vi "Initialize Tx Transfers.vi"(8 "error in (no error)":errorcluster, 10 "Tx Transfer configurations":T2[](array[typedef]) {"channels"."string offset" format="%d bytes"}, 11 "UDP Transceiver in":refnum<class "UDP Transceiver.lvclass">) -> (0 "error out":errorcluster, 1 "max buffer size":u64, 2 "Tx Transfer parameters":T1[](array[typedef]), 3 "UDP Transceiver out":refnum<class "UDP Transceiver.lvclass">)   [LabVIEW 2017, in "UDP.lvlib" / "UDP Transceiver.lvclass"]
uses:
  UDP Transceiver.lvclass
  Builds/Data Sharing Framework/Current/Core/DSF Core.lvlibp/Typedefs/DSF Engine Transfer Configuration.ctl
  Builds/Data Sharing Framework/Current/Core/DSF Core.lvlibp/Typedefs/DSF Byte Order.ctl
  Builds/Data Sharing Framework/Current/Core/DSF Core.lvlibp/Typedefs/DSF Settings Info.ctl
  Builds/Data Sharing Framework/Current/Core/DSF Core.lvlibp/Typedefs/DSF Engine Channel Configuration.ctl
  Builds/Data Sharing Framework/Current/Core/DSF Core.lvlibp/Typedefs/DSF Data Type.ctl
  Transfer Tx Parameters.ctl
  Builds/Data Sharing Framework/Current/Core/DSF Core.lvlibp/Typedefs/DSF Buffer Type.ctl
  UDP Transceiver.lvclass/UDP Transceiver.ctl
  Builds/Data Sharing Framework/Current/Core/DSF Core.lvlibp/Classes/Configuration/Required Buffer Size (Transfer).vi
  UDP Invalid Setting.vi
  Builds/Data Sharing Framework/Current/Core/DSF Core.lvlibp/Classes/Configuration/Configuration Session.lvclass
  Builds/Data Sharing Framework/Current/Core/DSF Core.lvlibp
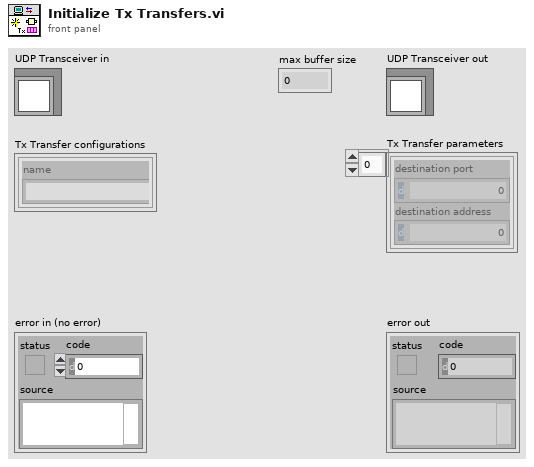
[diagram p1: front panel]
types:
  T1 = typedef "UDP.lvlib/UDP Transceiver.lvclass/Transfer Tx Parameters.ctl" = cluster{"destination port":u16, "destination address":u32}
  T2 = typedef "DSF Core.lvlibp/DSF Engine Transfer Configuration.ctl" = cluster{"name":string, "byte order":T3, "settings":T4, "channels":T5[]}
  T3 = typedef "DSF Core.lvlibp/DSF Byte Order.ctl" = enum8{"big-endian", "little-endian"}
  T4 = typedef "DSF Core.lvlibp/DSF Settings Info.ctl" = cluster{"component":string, "name":string, "values":cluster{"key":string, "value":string}[]}[]
  T5 = typedef "DSF Core.lvlibp/DSF Engine Channel Configuration.ctl" = cluster{"string offset":u64, "name":string, "units":string, "engine data type":T6, "string data type":T6, "settings":T4}
  T6 = typedef "DSF Core.lvlibp/DSF Data Type.ctl" = enum8{"Bool", "SGL", "DBL", "I8", "I16", "I32", "I64", "U8", "U16", "U32", "U64"}
  T7 = typedef "DSF Core.lvlibp/DSF Buffer Type.ctl" = enum16{"Engine", "String"}
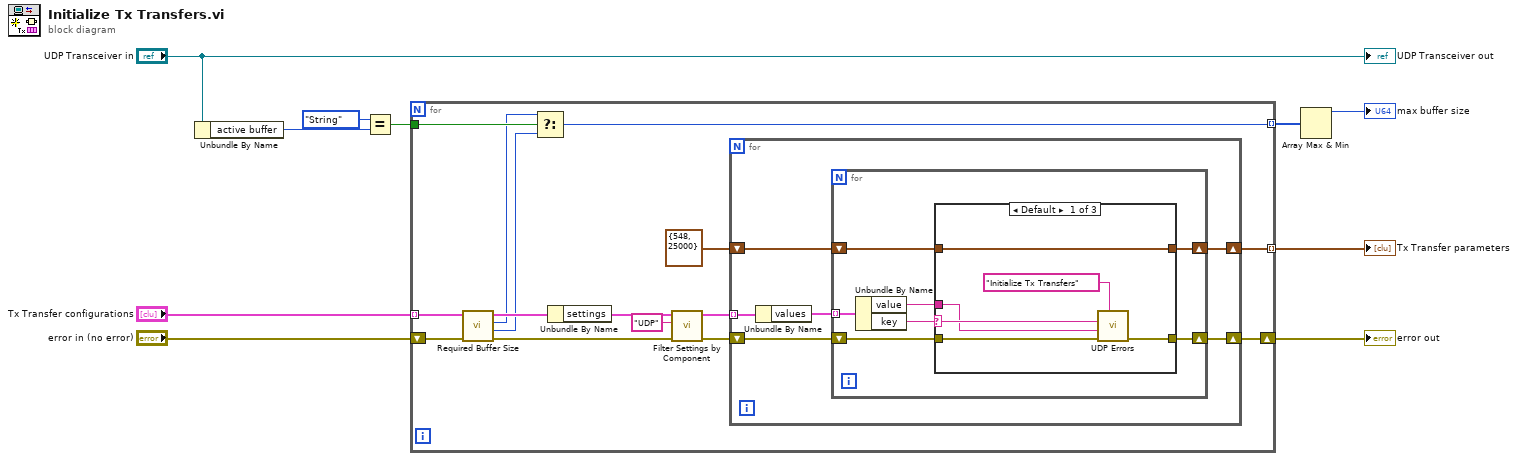
[diagram p0: block diagram]
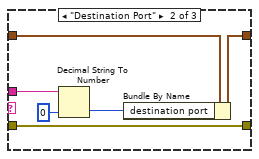
[diagram p2: hidden frame]
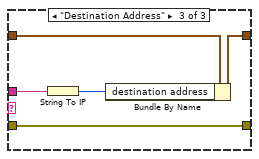
[diagram p3: hidden frame]
diagram:
  n1 = Unbundle By Name("UDP Transceiver in") -> ("active buffer"=w3:T7)
  n2 = Equal?(x=DSF_Buffer_Type."String", y=w3) -> (x = y?=w1:bool)
  n3 = for {
    shift-right: [w25] -> w7
    shift-left: "error in (no error)" -> [w22]
    tunnel: "Tx Transfer configurations" -> [w23] mode=indexing
    tunnel: [w24] -> w8 mode=indexing
    tunnel: [w12] -> w6 mode=indexing
    tunnel: w1 -> [w15]
    n4 = call-poly "Required Buffer Size.vi"("error in (no error)"=w22, "Transfer Configuration in"=w23) -> ("error out"=w20:errorcluster, "engine buffer size"=w14:u64, "string buffer size"=w13:u64, "Transfer Configuration out"=w21:T2)  [unwired: 6 in]
    n5 = Select(t=w13, s=w15, f=w14) -> (s? t:f=w12:u64)
    n6 = Unbundle By Name(w21) -> ("settings"=w16:T4)
    n7 = call "Filter Settings by Component.vi"("error in (no error)"=w20, "component"="UDP", "settings"=w16) -> ("error out"=w19:errorcluster, "filtered settings"=w17:T4)  [unwired: 7 in]
    n8 = for {
      tunnel: w17 -> [w27] mode=indexing
      shift-right: [w29] -> w24
      shift-left: T1 {"destination port"=548, "destination address"=25000} ("Transfer Tx") -> [w30]
      shift-right: [w31] -> w25
      shift-left: w19 -> [w28]
      n9 = Unbundle By Name(w27) -> ("values"=w26:cluster{"key":string, "value":string}[])
      n10 = for {
        tunnel: w26 -> [w38] mode=indexing
        shift-right: [w32] -> w31
        shift-left: w28 -> [w37]
        shift-right: [w35] -> w29
        shift-left: w30 -> [w36]
        n11 = Unbundle By Name(w38) -> ("value"=w33:string, "key"=w34:string)
        n12 = case shown="Default" w34 {
          selector: w34 -> [w40 _ _]
          tunnel: w33 -> [w39 w50 w54]
          tunnel: w37 -> [w42 w47 w55]
          tunnel: [w41 w47 w55] -> w32
          tunnel: w36 -> [w44 w46 w52]
          tunnel: [w44 w45 w51] -> w35
          frame Default {
            n13 = call-poly "UDP Errors.vi"("source vi name"="Initialize Tx Transfers", "error in (no error)"=w42, "value"=w39, "key"=w40) -> ("error out"=w41:errorcluster)  [unwired: 6 in, 1 out]
          }
          frame "Destination Port" {
            n14 = Decimal String To Number(string=w50, default (0L)=u16 0 ("default (0 I32)")) -> (number=w48:u16)  [unwired: 1 in, 1 out]
            n15 = Bundle By Name(cluster=w46, "destination port"=w48) -> (w45:T1)
          }
          frame "Destination Address" {
            n16 = String To IP(1:w54) -> (0:w53:u32)
            n17 = Bundle By Name(cluster=w52, "destination address"=w53) -> (w51:T1)
          }
        }
      }
    }
  }
  "error out" <- w7
  "Tx Transfer parameters" <- w8
  n18 = Array Max & Min(array=w6) -> (max value=→"max buffer size":u64)  [unwired: 3 out]
  "UDP Transceiver out" <- "UDP Transceiver in"
